vi "Destroy.vi"(8 "error in (no error)":errorcluster, 11 "Menu Item ref":refnum<data-value>) -> (0 "error out":errorcluster)   [LabVIEW 2016, in "MGI_MenuItem.lvclass"]
doc: "Destroys the MenuItem. This ensures that all references contained by the menu item are also destroyed. Do not use the \"Delete Data Value Reference\" on a MenuItem Reference as this will lead to memory leaks. Use this vi instead.\n\nAuthored by Derek E. Trepanier\nsupport@mooregoodideas.com\nwww.mooregoodideas.com\n\nCopyright (c) 2012, Moore Good Ideas, Inc.\n\nAll rights reserved.\n\nRedistribution and use in source and binary forms, with or without modification, are permitted provided that the following conditions are met:\n\n * Redistributions of source code must retain the above copyright notice, this list of conditions and the following disclaimer.\n * Redistributions in binary form must reproduce the above copyright notice, this list of conditions and the following disclaimer in the documentation and/or other materials provided with the distribution.\n * Neither the name of Moore Good Ideas, Inc. nor the names of its contributors may be used to endorse or promote products derived from this software without specific prior written permission.\n\nTHIS SOFTWARE IS PROVIDED BY THE COPYRIGHT HOLDERS AND CONTRIBUTORS \"AS IS\" AND ANY EXPRESS OR IMPLIED WARRANTIES, INCLUDING, BUT NOT LIMITED TO, THE IMPLIED WARRANTIES OF MERCHANTABILITY AND FITNESS FOR A PARTICULAR PURPOSE ARE DISCLAIMED. IN NO EVENT SHALL THE COPYRIGHT OWNER OR CONTRIBUTORS BE LIABLE FOR ANY DIRECT, INDIRECT, INCIDENTAL, SPECIAL, EXEMPLARY, OR CONSEQUENTIAL DAMAGES (INCLUDING, BUT NOT LIMITED TO, PROCUREMENT OF SUBSTITUTE GOODS OR SERVICES; LOSS OF USE, DATA, OR PROFITS; OR BUSINESS INTERRUPTION) HOWEVER CAUSED AND ON ANY THEORY OF LIABILITY, WHETHER IN CONTRACT, STRICT LIABILITY, OR TORT (INCLUDING NEGLIGENCE OR OTHERWISE) ARISING IN ANY WAY OUT OF THE USE OF THIS SOFTWARE, EVEN IF ADVISED OF THE POSSIBILITY OF SUCH DAMAGE."
uses:
  <userlib>/_MGI/Menu Building/MenuItem/MGI_MenuItem.lvclass
  <userlib>/_MGI/Menu Building/MenuItem/Read Sub-Menus.vi
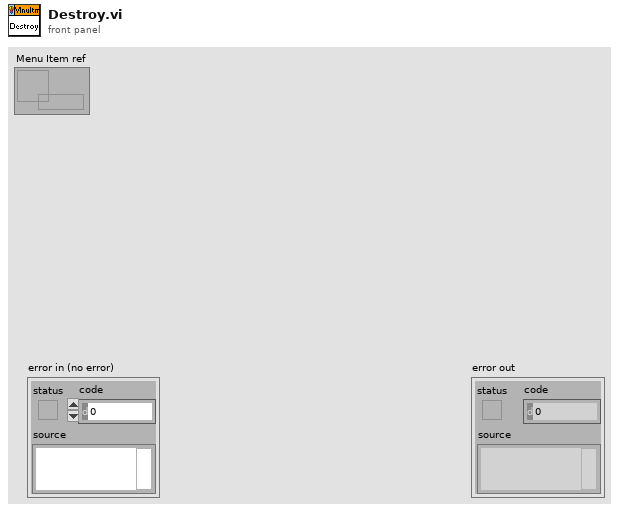
[diagram p1: front panel]
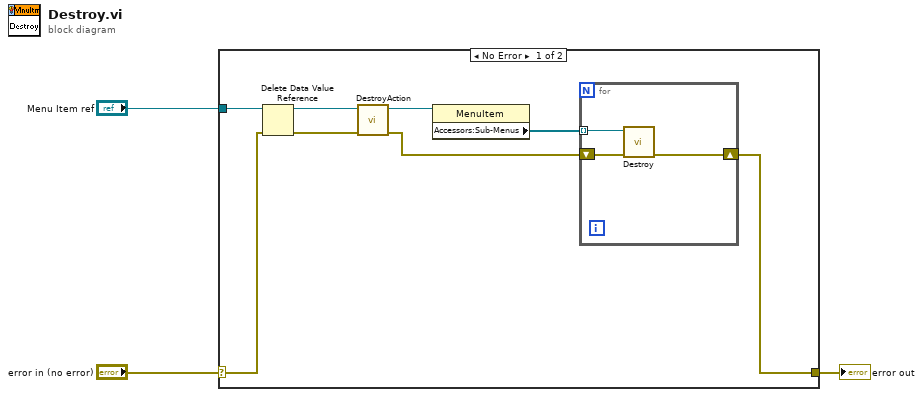
[diagram p0: block diagram]
diagram:
  n1 = case shown="No Error" "error in (no error)" {
    selector: "error in (no error)" -> [w10 w15]
    tunnel: [w4 w15] -> w1
    tunnel: "Menu Item ref" -> [w11 _]
    frame No Error {
      n2 = Delete Data Value Reference(data value reference=w11, error in=w10) -> (data value=w8:refnum<class "MGI_MenuItem.lvclass">, error out=w9:errorcluster)
      n3 = call-dynamic "DestroyAction.vi"("error in (no error)"=w9, "MenuItem in"=w8) -> ("error out"=w5:errorcluster, "MenuItem out"=w7:refnum<class "MGI_MenuItem.lvclass">)  [unwired: 8 in]
      n4 = property class="MenuItem"(reference=w7) -> ("Accessors:Sub-Menus"=w6:refnum<data-value>[])  [unwired: 1 in, 2 out]
      n5 = for {
        tunnel: w6 -> [w14] mode=indexing
        shift-right: [w12] -> w4
        shift-left: w5 -> [w13]
        n6 = call <userlib>:"Destroy.vi"("error in (no error)"=w13, "Menu Item ref"=w14) -> ("error out"=w12:errorcluster)  [unwired: 9 in]
      }
    }
    frame Error {
    }
  }
  "error out" <- w1
